vi "Run_Core.vi"(0 "Comparison Operations in":refnum<class "Comparison Operations.lvclass">, 11 "error in (no error)":errorcluster) -> (4 "Comparison Operations out":refnum<class "Comparison Operations.lvclass">, 6 "Return":variant, 15 "error out":errorcluster)   [LabVIEW 2016, in "Comparison Operations.lvclass"]
uses:
  Comparison Operations.lvclass
  D:/TOOLS/LSL/source code/LSL components/functions/functionsbase/functionbase.lvclass
  functionsbase/functionbase.lvclass/functionbase.ctl
  Comparison Operations.lvclass/Comparison Operations.ctl
  functionsbase/properties/Read Smart Syntax Representation.vi
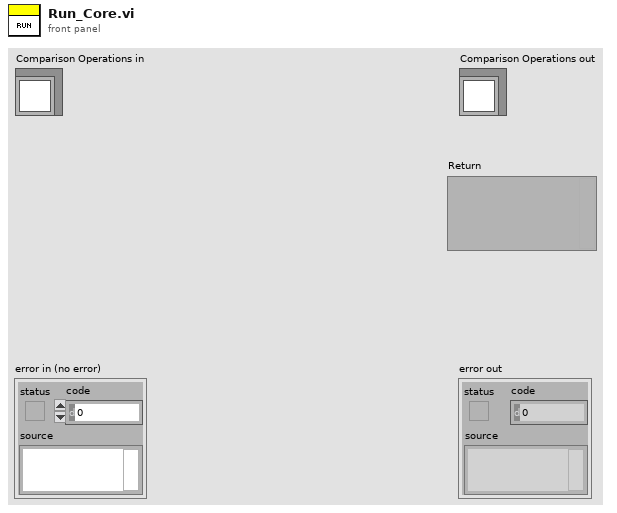
[diagram p1: front panel]
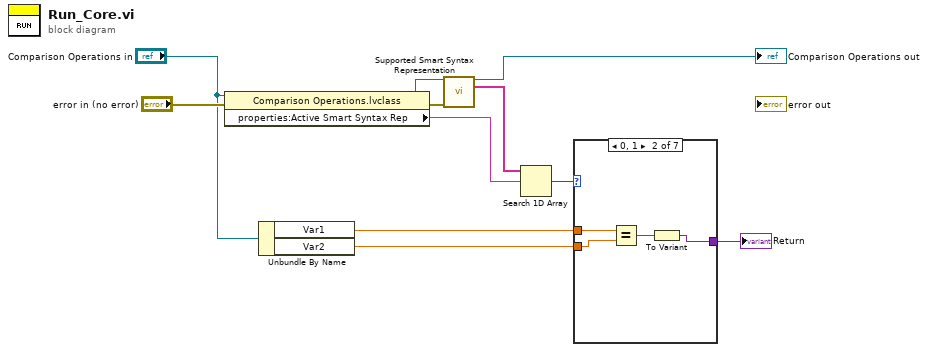
[diagram p0: block diagram]
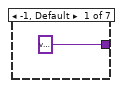
[diagram p2: hidden frame]
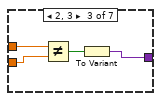
[diagram p3: hidden frame]
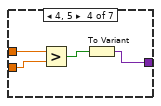
[diagram p4: hidden frame]
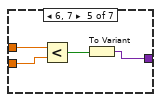
[diagram p5: hidden frame]
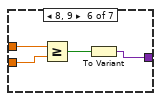
[diagram p6: hidden frame]
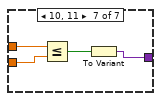
[diagram p7: hidden frame]
diagram:
  n1 = property class="Comparison Operations.lvclass"(reference="Comparison Operations in", error in="error in (no error)") -> (reference out=w7:refnum<class "Comparison Operations.lvclass">, error out=w10:errorcluster, "properties:Active Smart Syntax Rep"=w4:string)
  n2 = Unbundle By Name("Comparison Operations in") -> ("Var1"=w3:dbl, "Var2"=w2:dbl)
  n3 = call-dynamic "Supported Smart Syntax Representation.vi"("Comparison Operations in"=w7, "error in (no error)"=w10) -> ("Comparison Operations out"=→"Comparison Operations out":refnum<class "Comparison Operations.lvclass">, "Smart Syntax Representation List"=w9:string[])  [unwired: 11 in, 1 out]
  n4 = Search 1D Array(1D array=w9, element=w4) -> (index of element=w8:i32)  [unwired: 1 in]
  n5 = case shown="0, 1" w8 {
    tunnel: w3 -> [_ w14 w19 w22 w27 w32 w36]
    tunnel: w2 -> [_ w13 w18 w21 w26 w31 w35]
    tunnel: [variant ("Variant") w16 w20 w24 w28 w29 w33] -> w1
    frame -1, Default {
    }
    frame 0, 1 {
      n6 = Equal?(x=w14, y=w13) -> (x = y?=w15:bool)
      n7 = To Variant(anything=w15) -> (Variant=w16:variant)
    }
    frame 2, 3 {
      n8 = Not Equal?(x=w19, y=w18) -> (x != y?=w17:bool)
      n9 = To Variant(anything=w17) -> (Variant=w20:variant)
    }
    frame 4, 5 {
      n10 = Greater?(x=w22, y=w21) -> (0:w23:bool)
      n11 = To Variant(anything=w23) -> (Variant=w24:variant)
    }
    frame 6, 7 {
      n12 = Less?(x=w27, y=w26) -> (x < y?=w25:bool)
      n13 = To Variant(anything=w25) -> (Variant=w28:variant)
    }
    frame 8, 9 {
      n14 = Greater Or Equal?(x=w32, y=w31) -> (x >= y?=w30:bool)
      n15 = To Variant(anything=w30) -> (Variant=w29:variant)
    }
    frame 10, 11 {
      n16 = Less Or Equal?(x=w36, y=w35) -> (x <= y?=w34:bool)
      n17 = To Variant(anything=w34) -> (Variant=w33:variant)
    }
  }
  "Return" <- w1
